vi "Data Storage Thurough Reference.vi"(9 "Time Out In ms":i32=-1, 10 "Data In":u16[](array[numeric]), 11 "DVR In":refnum<data-value>) -> (1 "Time Out":bool, 3 "DVR Out":refnum<data-value>)   [LabVIEW 2019, in "Circular Buffer 1D U16 DVR Queue.lvclass"]
uses:
  Circular Buffer 1D U16 DVR Queue.lvclass
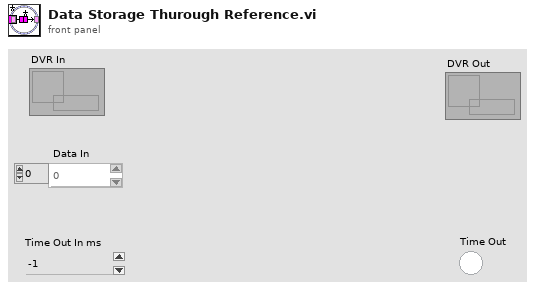
[diagram p1: front panel]
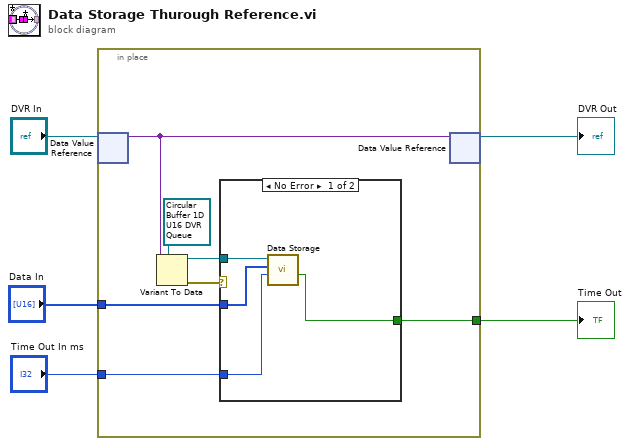
[diagram p0: block diagram]
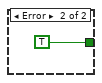
[diagram p2: hidden frame]
diagram:
  n1 = in-place {
    in-place-border: "Time Out In ms" -> [w8]
    in-place-border: [w7] -> w2
    in-place-border: "Data In" -> [w6]
    n2 = in-place-dvr #1("DVR In") -> (w11:variant)  [unwired: 1 out]
    n3 = Variant To Data(type=refnum<class "Circular Buffer 1D U16 DVR Queue.lvclass"> refnum ("Circular Buffer 1D U16 DVR Queue.lvclass"), Variant=w11) -> (data=w9:refnum<class "Circular Buffer 1D U16 DVR Queue.lvclass">, error out=w10:errorcluster)  [unwired: 1 in]
    n4 = case shown="No Error" w10 {
      tunnel: w9 -> [w16 _]
      tunnel: w8 -> [w14 _]
      tunnel: [w13 TRUE ("Time Out")] -> w7
      tunnel: w6 -> [w15 _]
      frame No Error {
        n5 = call "Data Storage.vi"("Time Out In ms"=w14, "Data In"=w15, "Circular Buffer 1D U16 DVR Queue in"=w16) -> ("Time Out"=w13:bool)  [unwired: 7 in, 1 out]
      }
      frame Error {
      }
    }
    n6 = in-place-dvr #1(w11) -> (→"DVR Out":refnum<data-value>)  [unwired: 1 out]
  }
  "Time Out" <- w2
